vi "Loop (Data Stream).vi"(8 "Error IN":errorcluster, 11 "Stop":refnum<vi>) -> (0 "Error OUT":errorcluster)   [LabVIEW 2019]
uses:
  Controls/Stream TCP Data Stream Mode (RT).ctl
  Controls/Stream RT FIFO Mode.ctl
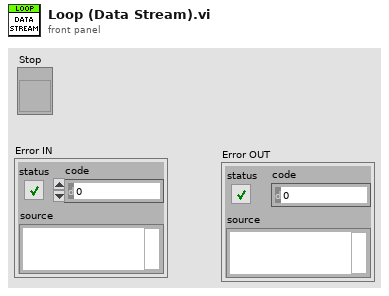
[diagram p1: front panel]
types:
  T1 = typedef "Stream TCP Data Stream Mode (RT).ctl" = enum16{"Init", "Write Data", "Close"}
  T2 = typedef "Stream RT FIFO Mode.ctl" = enum16{"Create", "Write", "Read", "Delete"}
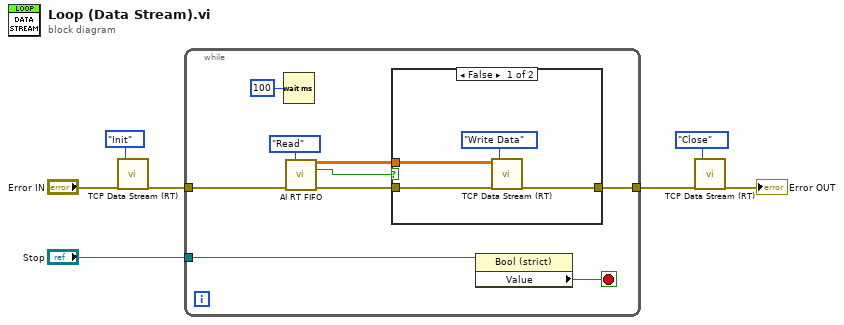
[diagram p0: block diagram]
diagram:
  n1 = call "TCP Data Stream (RT).vi"("Error IN"="Error IN", "Mode"=Stream_TCP_Data_Stream_Mode_(RT)."Init") -> ("Error OUT"=w7:errorcluster)  [unwired: 16 in, 1 out]
  n2 = while {
    tunnel: w7 -> [w16]
    tunnel: [w14] -> w2
    tunnel: "Stop" -> [w10]
    stop <- w11 stop-if-true
    n3 = Wait (ms)(milliseconds to wait=u32 100) -> ()  [unwired: 1 out]
    n4 = call "AI RT FIFO.vi"("Mode"=Stream_RT_FIFO_Mode."Read", "Error IN"=w16) -> ("Data OUT"=w12:dbl[][], "Empty?"=w15:bool, "Error OUT"=w13:errorcluster)  [unwired: 11 in]
    n5 = case shown="False" w15 {
      tunnel: w12 -> [w19 _]
      tunnel: [w17 w21] -> w14
      tunnel: w13 -> [w18 w21]
      frame False {
        n6 = call "TCP Data Stream (RT).vi"("Data"=w19, "Error IN"=w18, "Mode"=Stream_TCP_Data_Stream_Mode_(RT)."Write Data") -> ("Error OUT"=w17:errorcluster)  [unwired: 15 in, 1 out]
      }
      frame True {
      }
    }
    n7 = property class="Bool (strict)"(reference=w10) -> ("Value"=w11:bool)  [unwired: 1 in, 2 out]
  }
  n8 = call "TCP Data Stream (RT).vi"("Error IN"=w2, "Mode"=Stream_TCP_Data_Stream_Mode_(RT)."Close") -> ("Error OUT"=→"Error OUT":errorcluster)  [unwired: 16 in, 1 out]
